vi "myRIO v1.0 Reserve DI Block.vi"(7 "Allow multiple opens?":bool, 8 "error in (no error)":errorcluster, 10 "DI (N Samples) Channel List":T2, 11 "Generic FPGA Reference":T1) -> (0 "error out":errorcluster)   [LabVIEW 2021]
uses:
  <vilib>/myRIO/Common/Instrument Driver Framework/myRIO v1.0/DI Block/typedefs/DI Block Channels List.ctl
  <vilib>/myRIO/Common/Instrument Driver Framework/myRIO v1.0/DI Block/typedefs/DI Block Channels Enum.ctl
  <vilib>/myRIO/Common/Instrument Driver Framework/Utilities/typedefs/Generic FPGA Reference.ctl
  <vilib>/myRIO/Common/Instrument Driver Framework/myRIO v1.0/DI Block/typedefs/DI Block FPGA Reference.ctl
  <vilib>/myRIO/Common/Instrument Driver Framework/myRIO v1.0/Resource Manager/vis/myRIO v1.0 Reserve Channel.vi
  <vilib>/myRIO/Common/Instrument Driver Framework/myRIO v1.0/Resource Manager/vis/myRIO v1.0 Unreserve Channel.vi
  <vilib>/myRIO/Common/Instrument Driver Framework/myRIO v1.0/Resource Manager/vis/myRIO v1.0 Build Mutex Name.vi
  <vilib>/myRIO/Common/Instrument Driver Framework/myRIO v1.0/Resource Manager/vis/myRIO v1.0 Block Write Configuration.vi
  <vilib>/myRIO/Common/Instrument Driver Framework/Utilities/vis/IO Manager.vi
  <vilib>/Utility/error.llb/Error Cluster From Error Code.vi
  <vilib>/myRIO/Common/Instrument Driver Framework/Utilities/vis/Configuration Manager.vi
  <vilib>/rvi/interface/common/niFpgaWaitOnOcc.vi
  <vilib>/rvi/interface/nirviMethod/nirviMethod.xnode
  <vilib>/FPGAPlugInAG/Dynamic/niLvFpga_ConfigureFifo_Dynamic.vi
  <vilib>/rvi/errors/niLvFpgaMergeErrorWithErrorCode.vi
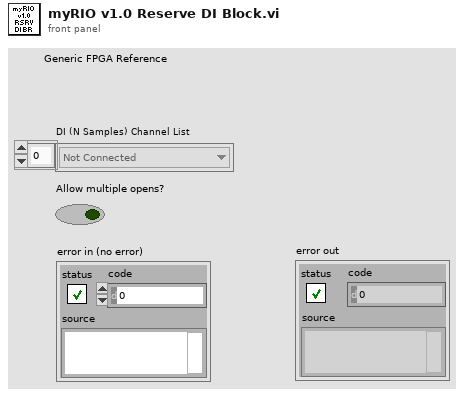
[diagram p1: front panel]
types:
  T1 = typedef "Generic FPGA Reference.ctl" = refnum<k20>
  T2 = typedef "DI Block Channels List.ctl" = T3[]
  T3 = typedef "DI Block Channels Enum.ctl" = enum16{"Not Connected", "A/DI0 (N Samples)", "A/DI1 (N Samples)", "A/DI2 (N Samples)", "A/DI3 (N Samples)", "A/DI4 (N Samples)", "A/DI5 (N Samples)", "A/DI6 (N Samples)", "A/DI7 (N Samples)", "A/DI8 (N Samples)", "A/DI9 (N Samples)", "A/DI10 (N Samples)", "A/DI11 (N Samples)", "A/DI12 (N Samples)", "A/DI13 (N Samples)", "A/DI14 (N Samples)", "A/DI15 (N Samples)", "A/DI16 (N Samples)", "A/DI17 (N Samples)", "A/DI18 (N Samples)", "A/DI19 (N Samples)", "B/DI0 (N Samples)", "B/DI1 (N Samples)", "B/DI2 (N Samples)", "B/DI3 (N Samples)", "B/DI4 (N Samples)", "B/DI5 (N Samples)", "B/DI6 (N Samples)", "B/DI7 (N Samples)", "B/DI8 (N Samples)", "B/DI9 (N Samples)", "B/DI10 (N Samples)", "B/DI11 (N Samples)", "B/DI12 (N Samples)", "B/DI13 (N Samples)", "B/DI14 (N Samples)", "B/DI15 (N Samples)", "B/DI16 (N Samples)", "B/DI17 (N Samples)", "B/DI18 (N Samples)", "B/DI19 (N Samples)"}
  T4 = typedef "DI Block FPGA Reference.ctl" = refnum<k20>
  T5 = typedef "myRIO v1.0 Channel Reservation List.ctl" = T6[]
  T6 = typedef "myRIO v1.0 Channel Reservation Info.ctl" = cluster{"Channel Name":string, "Connector":T7, "Mutex ID":i32}
  T7 = typedef "myRIO v1.0 Connector List.ctl" = enum32{"None", "ConnectorA", "ConnectorB", "ConnectorC"}
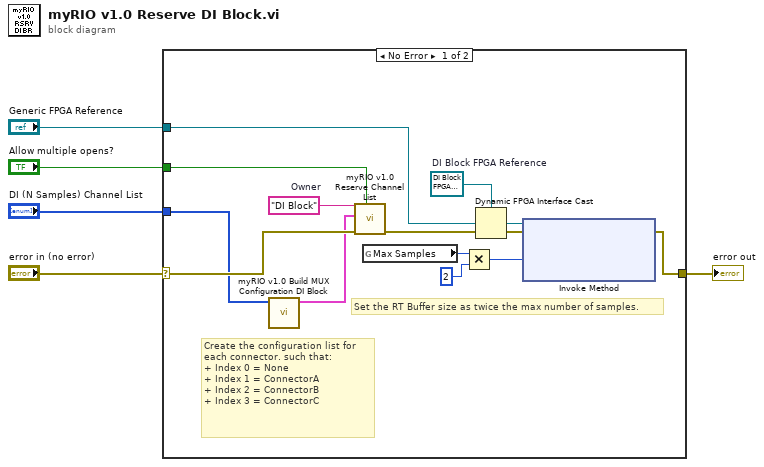
[diagram p0: block diagram]
diagram:
  n1 = case shown="No Error" "error in (no error)" {
    selector: "error in (no error)" -> [w17 w19]
    tunnel: "DI (N Samples) Channel List" -> [w14 _]
    tunnel: [w6 w19] -> w4
    tunnel: "Allow multiple opens?" -> [w18 _]
    tunnel: "Generic FPGA Reference" -> [w13 _]
    frame No Error {
      w12 = T4 refnum  # DI Block FPGA Reference
      w16 = "DI Block"  # Owner
      # "Create the configuration list for each connector. such that:\n+ Index 0 = None\n+ Index 1 = ConnectorA\n+ Index 2 = ConnectorB \n+ Index 3 = ConnectorC"
      # "Set the RT Buffer size as twice the max number of samples."
      n2 = call <vilib>:"myRIO v1.0 Build MUX Configuration DI Block.vi"("DI (N Samples) Channel List"=w14) -> ("Channel Reservation List"=w15:T5)  [unwired: 10 in]
      n3 = call <vilib>:"myRIO v1.0 Reserve Channel List.vi"("Allow multiple opens?"=w18, "error in (no error)"=w17, "Channel Reservation List"=w15, "Owner"=w16) -> ("error out"=w8:errorcluster)  [unwired: 7 in]
      n4 = global read "myRIO v1.0 Block Write Configuration.vi" "Max Samples"() -> (w11:u32)
      n5 = Multiply(x=w11, y=u32 2) -> (x*y=w7:u32)
      n6 = Dynamic FPGA Interface Cast(Session In=w12, Type=w13) -> (Session Out=w9:T4)
      n7 = xnode "Invoke Method"("FPGA VI Reference In"=w9, "error in"=w8, "Requested Depth"=w7) -> ("error out"=w6:errorcluster)  [unwired: 2 out]
    }
    frame Error {
    }
  }
  "error out" <- w4
